vi "File,Check if Dir is in List.vi"(10 "Path":path, 11 "List of Paths":path[](array[path])) -> (2 "Index":i32, 3 "In List":bool)   [LabVIEW 2024, in "EQMF.lvlib" / "File Utils.lvlib"]
uses:
  File Utils.lvlib
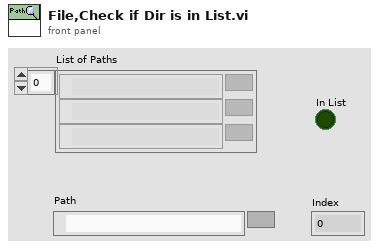
[diagram p1: front panel]
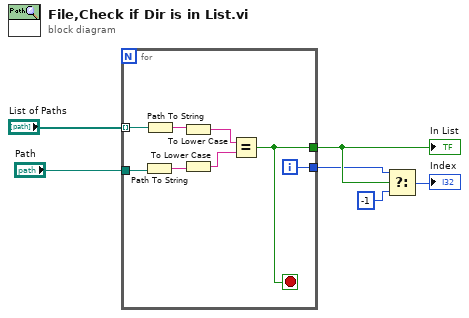
[diagram p0: block diagram]
diagram:
  n1 = for {
    tunnel: "List of Paths" -> [w14] mode=indexing
    tunnel: "Path" -> [w13]
    tunnel: [w8] -> w3
    tunnel: [w7] -> w1
    i -> [w7]
    stop <- w8 stop-if-true
    n2 = Path To String(path=w13) -> (string=w11:string)
    n3 = Path To String(path=w14) -> (string=w12:string)
    n4 = To Lower Case(string=w12) -> (all lower case string=w10:string)
    n5 = To Lower Case(string=w11) -> (all lower case string=w9:string)
    n6 = Equal?(x=w10, y=w9) -> (x = y?=w8:bool)
  }
  "In List" <- w3
  n7 = Select(t=w1, s=w3, f=-1) -> (s? t:f=→"Index":i32)
